vi "Processed Data Handler.vi"(8 "error in":errorcluster, 9 "Processed Data Notifier":refnum<notifier>, 11 "Data":T1) -> (0 "error out":errorcluster)   [LabVIEW 2024]
uses:
  support/Control/Array Data Constant.ctl
  support/Control/Data Constant.ctl
  <vilib>/Analysis/baseanly.llb/Mean (DBL).vi
  <vilib>/Analysis/NI_AALBase.lvlib
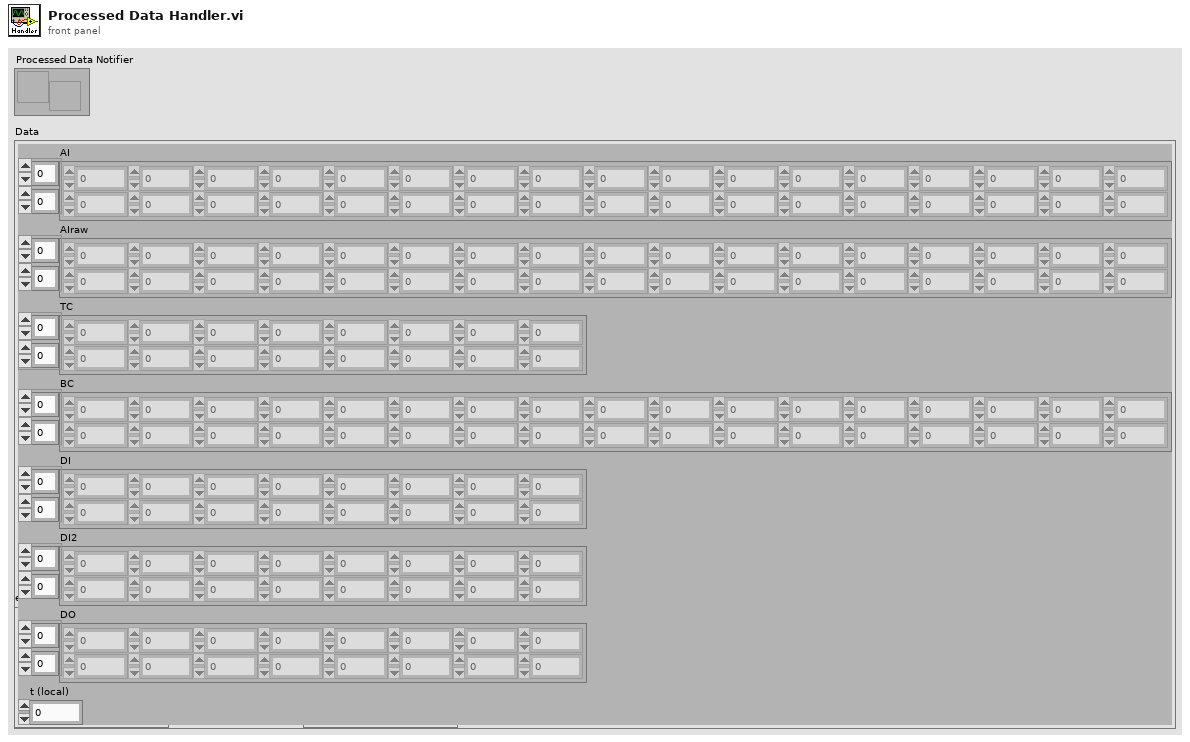
[diagram p1: front panel]
types:
  T1 = typedef "Data Constant.ctl" = cluster{"AI":dbl[][], "AIraw":dbl[][], "TC":dbl[][], "BC":dbl[][], "DI":dbl[][], "DI2":dbl[][], "DO":dbl[][], "t (local)":dbl}
  T2 = typedef "Array Data Constant.ctl" = cluster{"AI":dbl[], "TC":dbl[], "BC":dbl[], "DI":dbl[], "t (UTC)":dbl}
  T3 = typedef "LVDateTimeRec.ctl" = cluster{"fractional second":dbl, "second":i32, "minute":i32, "hour":i32, "day of month":i32, "month":i32, "year":i32, "day of week":i32, "day of year":i32, "DST":i32}
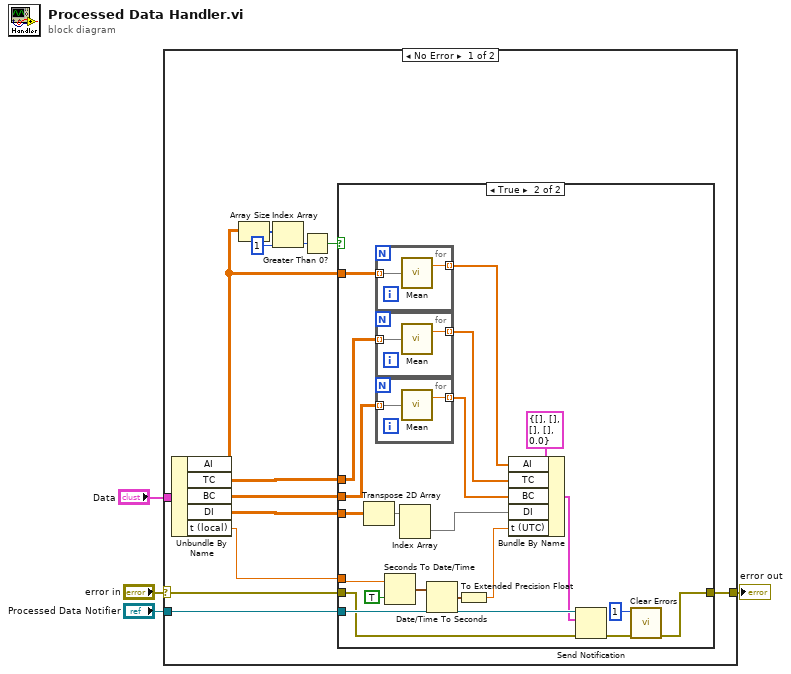
[diagram p0: block diagram]
diagram:
  n1 = case shown="No Error" "error in" {
    selector: "error in" -> [w16 w46]
    tunnel: [w11 w46] -> w3
    tunnel: "Processed Data Notifier" -> [w17 _]
    tunnel: "Data" -> [w15 _]
    frame No Error {
      n2 = Unbundle By Name(w15) -> ("AI"=w6:dbl[][], "TC"=w14:dbl[][], "BC"=w13:dbl[][], "DI"=w12:dbl[][], "t (local)"=w5:dbl)
      n3 = Array Size(array=w6) -> (size(s)=w10:i32[])
      n4 = Index Array(array=w10, index=1) -> (element=w9:i32)
      n5 = Greater Than 0?(x=w9) -> (x > 0?=w8:bool)
      n6 = case shown="True" w8 {
        tunnel: w17 -> [_ w39]
        tunnel: w16 -> [w18 w38]
        tunnel: w6 -> [_ w35]
        tunnel: w14 -> [_ w34]
        tunnel: w13 -> [_ w33]
        tunnel: w12 -> [_ w30]
        tunnel: [w18 w25] -> w11
        tunnel: w5 -> [_ w21]
        frame False {
        }
        frame True {
          n7 = Transpose 2D Array(2D array=w30) -> (transposed array=w28:dbl[][])
          n8 = for {
            tunnel: w35 -> [w45] mode=indexing
            tunnel: [w44] -> w19 mode=indexing
            n9 = call-poly <vilib>:"Mean.vi"("X"=w45) -> ("mean"=w44:dbl)  [unwired: 1 out]
          }
          n10 = for {
            tunnel: w34 -> [w43] mode=indexing
            tunnel: [w42] -> w31 mode=indexing
            n11 = call-poly <vilib>:"Mean.vi"("X"=w43) -> ("mean"=w42:dbl)  [unwired: 1 out]
          }
          n12 = for {
            tunnel: w33 -> [w41] mode=indexing
            tunnel: [w40] -> w32 mode=indexing
            n13 = call-poly <vilib>:"Mean.vi"("X"=w41) -> ("mean"=w40:dbl)  [unwired: 1 out]
          }
          n14 = Seconds To Date/Time(time stamp (now)=w21, to UTC (F)=TRUE) -> (date time rec=w23:T3)
          n15 = Index Array(array=w28) -> (element=w29:dbl[])  [unwired: 2 in]
          n16 = Date/Time To Seconds(2:w23) -> (0:w24:timestamp)  [unwired: 1 in]
          n17 = To Extended Precision Float(1:w24) -> (0:w20:ext)
          n18 = Bundle By Name(cluster=T2 {"AI"=[], "TC"=[], "BC"=[], "DI"=[], "t (UTC)"=0.0} ("Array Data Constant"), "AI"=w19, "TC"=w31, "BC"=w32, "DI"=w29, "t (UTC)"=w20) -> (w36:T2)
          n19 = Send Notification(notification=w36, notifier=w39, error in (no error)=w38) -> (error out=w27:errorcluster)  [unwired: 1 out]
          n20 = call <vilib>:"Clear Errors.vi"("error in (no error)"=w27, "specific error code to clear (0: all)"=1) -> ("error out"=w25:errorcluster)  [unwired: 4 in, 1 out]
        }
      }
    }
    frame Error {
    }
  }
  "error out" <- w3
